vi "Imaging event parser.vi"(8 "Imaging State in":T1, 11 "Status":T2 {"Setting"."X Pos." scale=-2.0..2.0; "Setting"."Y Pos." scale=-2.0..2.0}) -> (0 "Imaging State out":T1, 1 "last line?":bool, 2 "line #":i32, 4 "Data":string, 5 "Effective lines":dbl[][](array[numeric]))   [LabVIEW 2013]
uses:
  init & communication/init-status.ctl
  init & communication/Setting.ctl
  init & communication/event-package.ctl
  init & communication/Event1.ctl
  init & communication/data-package.ctl
  init & communication/Event.ctl
  Imaging State.ctl
panel:
  out "队列中元素数量":i32
  out "大小":i32
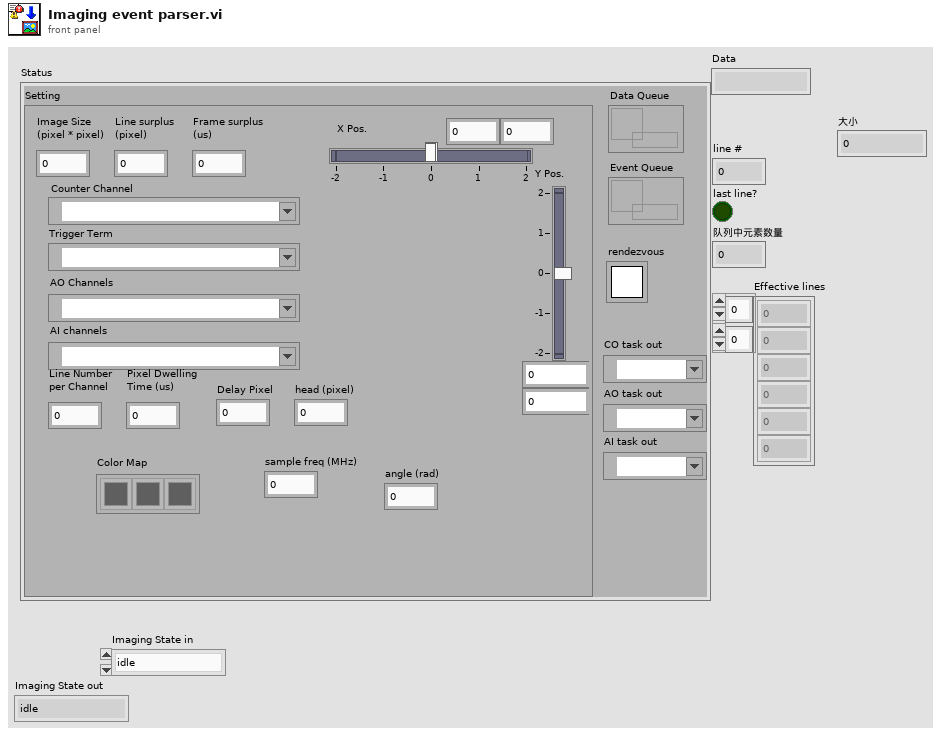
[diagram p1: front panel]
types:
  T1 = typedef "Imaging State.ctl" = enum16{"idle", "waiting for saving sheet", "waiting for stopping", "waiting for saving tiff", "init countinuous saving", "continuous saving", ""}
  T2 = typedef "init-status.ctl" = cluster{"Setting":T3, "Event Queue":refnum<queue>, "Data Queue":refnum<queue>, "rendezvous":T4, "CO task out":refnum<k21>, "AO task out":refnum<k21>, "AI task out":refnum<k21>}
  T3 = typedef "Setting.ctl" = cluster{"Image Size\n(pixel * pixel)":i32, "Counter Channel":tag, "Trigger Term":tag, "AO Channels":tag, "Y Pos.":cluster{dbl, dbl}, "X Pos.":cluster{dbl, dbl}, "Line surplus\n(pixel)":i32, "Frame surplus\n(us)":i32, "AI channels":tag, "Line Number\nper Channel":i32, "Delay Pixel":i32, "Pixel Dwelling\nTime (us)":i32, "Color Map":u32[], "head (pixel)":i32, "sample freq (MHz)":dbl, "angle (rad)":dbl}
  T4 = typedef "Rendezvous RefNum" = refnum<k1>
  T5 = typedef "event-package.ctl" = cluster{"Event":T6, "Data":string}
  T6 = typedef "Event1.ctl" = enum16{"null", "stop AI", "stop AO", "stop Imaging", "stop Counter", "save sheet", "restart", "save tiff", "gain/offset changed", "save multiple tiffs"}
  T7 = typedef "data-package.ctl" = cluster{"Event":T8, "Data":dbl[], "line #":i32}
  T8 = typedef "Event.ctl" = u16
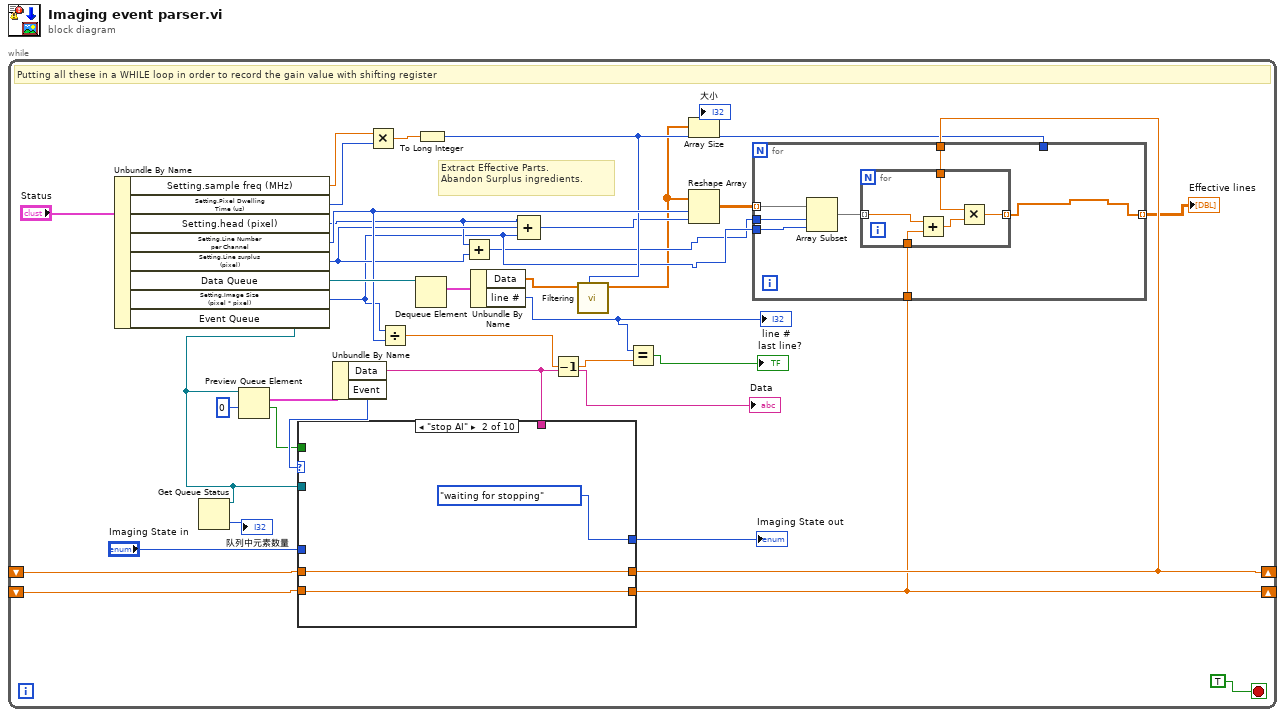
[diagram p0: block diagram]
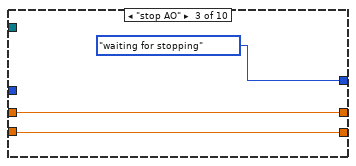
[diagram p3: hidden frame]
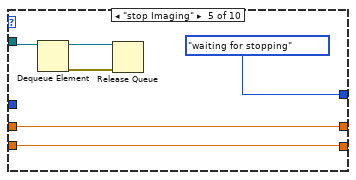
[diagram p5: hidden frame]
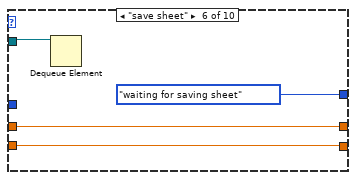
[diagram p6: hidden frame]
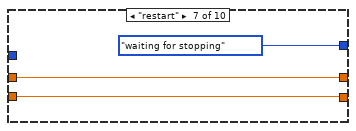
[diagram p7: hidden frame]
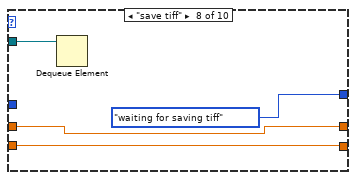
[diagram p8: hidden frame]
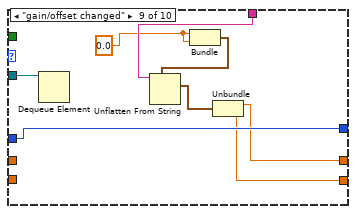
[diagram p9: hidden frame]
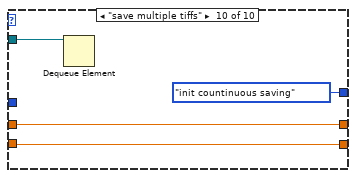
[diagram p10: hidden frame]
diagram:
  n1 = while {
    shift-right: [w18] -> _
    shift-left: _ -> [w17]
    shift-right: [w15] -> _
    shift-left: _ -> [w16]
    stop <- TRUE stop-if-true
    # "Extract Effective Parts.\nAbandon Surplus ingredients."
    # "Putting all these in a WHILE loop in order to record the gain value with shifting register"
    n2 = Unbundle By Name("Status") -> ("Setting.sample freq (MHz)"=w13:dbl, "Setting.Pixel Dwelling\nTime (us)"=w12:i32, "Setting.head (pixel)"=w21:i32, "Setting.Line Number\nper Channel"=w27:i32, "Setting.Line surplus\n(pixel)"=w22:i32, "Data Queue"=w34:refnum<queue>, "Setting.Image Size\n(pixel * pixel)"=w8:i32, "Event Queue"=w2:refnum<queue>)
    n3 = Get Queue Status(queue=w2) -> (# elements in queue=→"队列中元素数量":i32)  [unwired: 2 in, 7 out]
    n4 = Preview Queue Element(queue=w2, timeout in ms (-1)=0 ("超时毫秒(-1)")) -> (element=w30:T5, timed out?=w3:bool)  [unwired: 1 in, 2 out]
    n5 = Unbundle By Name(w30) -> ("Data"=w19:string, "Event"=w33:T6)
    "Data" <- w19
    n6 = case shown="\"stop AI\"" w33 {
      tunnel: "Imaging State in" -> [w51 _ _ w60 _ _ _ _ w84 _]
      tunnel: [w51 Imaging_State."waiting for stopping" ("Imaging State in") Imaging_State."waiting for stopping" ("Imaging State in") w60 Imaging_State."waiting for stopping" ("Imaging State in") Imaging_State."waiting for saving sheet" ("Imaging State in") Imaging_State."waiting for stopping" ("Imaging State in") Imaging_State."waiting for saving tiff" ("Imaging State in") w84 Imaging_State."init countinuous saving" ("Imaging State in")] -> w31
      tunnel: w2 -> [_ _ _ _ w63 w69 _ w77 w85 w89]
      tunnel: w19 -> [_ _ _ _ _ _ _ _ w83 _]
      tunnel: [w50 w54 w57 w59 w65 w68 w72 w75 w79 w87] -> w18
      tunnel: w17 -> [w50 w54 w57 w59 w65 w68 w72 w75 _ w87]
      tunnel: w16 -> [w49 w53 w56 w58 w64 w67 w71 w74 _ w86]
      tunnel: [w49 w53 w56 w58 w64 w67 w71 w74 w78 w86] -> w15
      tunnel: w3 -> [_ _ _ _ _ _ _ _ _ _]
      frame "null", Default {
      }
      frame "stop AI" {
      }
      frame "stop AO" {
      }
      frame "stop Counter" {
      }
      frame "stop Imaging" {
        n7 = Dequeue Element(queue=w63) -> (queue out=w62:refnum<queue>, error out=w61:errorcluster)  [unwired: 2 in, 2 out]
        n8 = Release Queue(queue=w62, error in (no error)=w61) -> ()  [unwired: 1 in, 3 out]
      }
      frame "save sheet" {
        n9 = Dequeue Element(queue=w69) -> ()  [unwired: 2 in, 4 out]
      }
      frame "restart" {
      }
      frame "save tiff" {
        n10 = Dequeue Element(queue=w77) -> ()  [unwired: 2 in, 4 out]
      }
      frame "gain/offset changed" {
        w82 = 0.0
        n11 = Dequeue Element(queue=w85) -> ()  [unwired: 2 in, 4 out]
        n12 = Bundle(w82, w82) -> (w81:cluster{dbl, dbl})  [unwired: 1 in]
        n13 = Unflatten From String(type=w81, binary string=w83) -> (value=w80:cluster{dbl, dbl})  [unwired: 3 in, 2 out]
        n14 = Unbundle(w80) -> (w79:dbl, w78:dbl)
      }
      frame "save multiple tiffs" {
        n15 = Dequeue Element(queue=w89) -> ()  [unwired: 2 in, 4 out]
      }
    }
    "Imaging State out" <- w31
    n16 = Multiply(x=w13, y=w12) -> (x*y=w11:dbl)
    n17 = Divide(x=w8, y=w27) -> (x/y=w23:dbl)
    n18 = Dequeue Element(queue=w34) -> (element=w35:T7)  [unwired: 2 in, 3 out]
    n19 = To Long Integer(number=w11) -> (32bit integer=w10:i32)
    n20 = Add(x=w21, y=w22) -> (x+y=w7:i32)
    n21 = Unbundle By Name(w35) -> ("Data"=w6:dbl[], "line #"=w25:i32)
    "line #" <- w25
    n22 = Compound Arithmetic op=ADD(w21, w22, w8) -> (w9:i32)
    n23 = Decrement(x=w23) -> (x-1=w24:dbl)
    n24 = call "Filtering.vi"("dwelling pixels"=w10, "数组输入"=w6) -> ("数组输出"=w4:dbl[])  [unwired: 9 in]
    n25 = Equal?(x=w25, y=w24) -> (x = y?=→"last line?":bool)
    n26 = Array Size(array=w4) -> (size(s)=→"大小":i32)
    n27 = Reshape Array(w4, w27, w9) -> (w28:dbl[][])
    n28 = for {
      tunnel: w28 -> [w43] mode=indexing
      tunnel: w7 -> [w42]
      tunnel: w8 -> [w41]
      tunnel: [w37] -> w14 mode=indexing
      tunnel: w18 -> [w39]
      tunnel: w15 -> [w38]
      tunnel: w10 -> [_]
      n29 = Array Subset(array=w43, index=w42, length=w41) -> (w40:dbl[])
      n30 = for {
        tunnel: w40 -> [w46] mode=indexing
        tunnel: w39 -> [w47]
        tunnel: [w48] -> w37 mode=indexing
        tunnel: w38 -> [w44]
        n31 = Add(x=w46, y=w44) -> (x+y=w45:dbl)
        n32 = Multiply(x=w47, y=w45) -> (x*y=w48:dbl)
      }
    }
    "Effective lines" <- w14
  }
